vi "Read all flows.vi"(0 "VISA resource name":refnum<visa-resource-name>="COM5") -> (11 "Flow 8":dbl, 13 "Flow 7":dbl, 14 "Flow 1":dbl, 15 "Flow 2":dbl, 16 "Flow 3":dbl, 17 "Flow 4":dbl, 18 "Flow 5":dbl, 19 "Flow 6":dbl)   [LabVIEW 2013]
uses:
  <vilib>/Instr/_visa.llb/VISA Configure Serial Port (Instr).vi
panel:
  out "GCF 8":dbl=1.0
  out "GCF 7":dbl=1.0
  out "GCF 6":dbl=1.0
  out "MFC 8 Size":dbl=1.0
  out "MFC 7 Size":dbl=1.0
  out "MFC 6 Size":dbl=1.0
  out "GCF 5":dbl=0.94
  out "GCF 4":dbl=1.47
  out "GCF 3":dbl=1.22
  out "GCF 2":dbl=0.9
  out "GCF 1":dbl=0.95
  out "MFC 5 Size":dbl=100.0
  out "MFC 4 Size":dbl=50.0
  out "MFC 3 Size":dbl=50.0
  out "MFC 2 Size":dbl=100.0
  out "MFC 1 Size":dbl=50.0
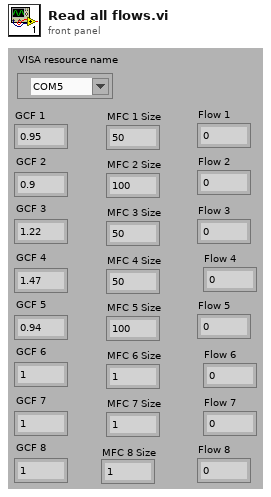
[diagram p1: front panel]
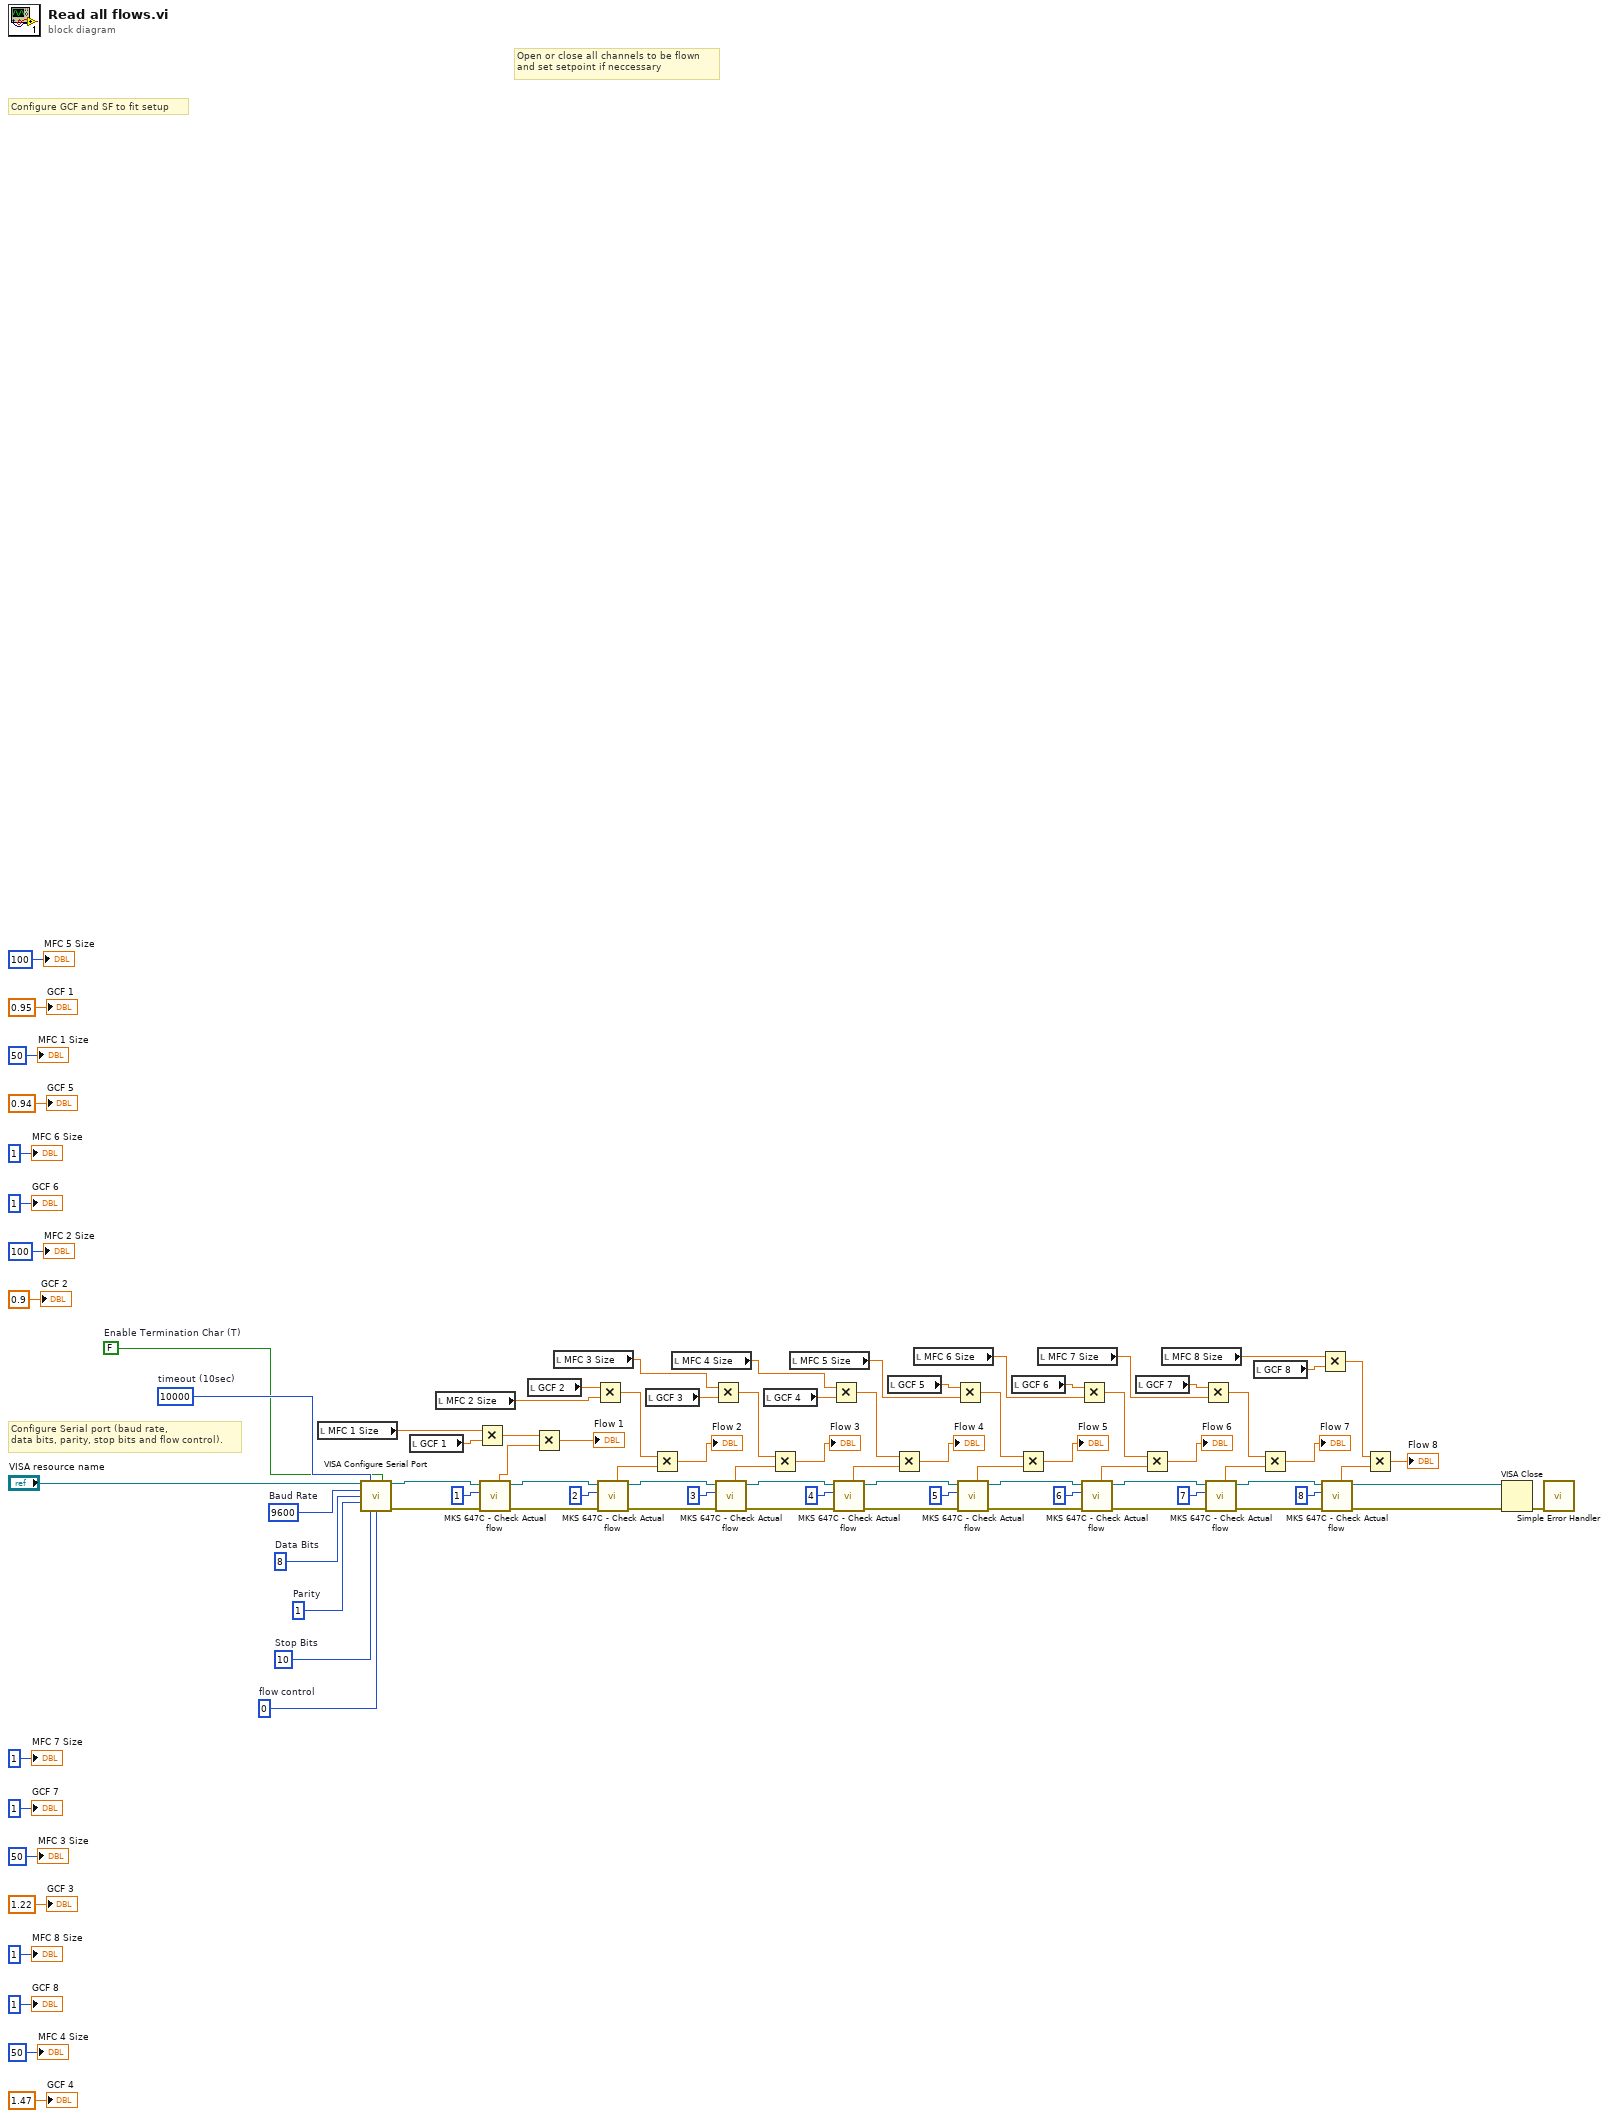
[diagram p0: block diagram]
diagram:
  w84 = 0  # flow control
  w85 = 10  # Stop Bits
  w86 = 1  # Parity
  w87 = 8  # Data Bits
  w88 = 9600  # Baud Rate
  w89 = FALSE  # Enable Termination Char (T)
  w90 = u32 10000  # timeout (10sec)
  # "Open or close all channels to be flown\nand set setpoint if neccessary"
  # "Configure GCF and SF to fit setup"
  # "Configure Serial port (baud rate,\ndata bits, parity, stop bits and flow control)."
  n1 = local read "MFC 1 Size"() -> (w61:dbl)
  n2 = call-poly "VISA Configure Serial Port"("VISA resource name"="VISA resource name", "timeout (10sec)"=w90, "Enable Termination\nChar (T)"=w89, "baud rate (9600)"=w88, "data bits (8)"=w87, "parity (0:none)"=w86, "stop bits (10: 1 bit)"=w85, "flow control (0:none)"=w84) -> ("VISA resource name out"=w66:refnum<visa-resource-name>, "error out"=w64:errorcluster)  [unwired: 6 in]
  n3 = local read "GCF 1"() -> (w60:dbl)
  n4 = local read "MFC 2 Size"() -> (w23:dbl)
  n5 = Multiply(x=w61, y=w60) -> (x*y=w63:dbl)
  n6 = call "MKS 647C - Check Actual flow.vi"("error in (no error)"=w64, "Channel"=1, "VISA resource name (IN)"=w66) -> ("error out"=w36:errorcluster, "VISA resource name (OUT)"=w37:refnum<visa-resource-name>, "Flow value"=w62:dbl)  [unwired: 6 in]
  n7 = local read "GCF 2"() -> (w22:dbl)
  n8 = Multiply(x=w63, y=w62) -> (x*y=→"Flow 1":dbl)
  n9 = local read "MFC 3 Size"() -> (w18:dbl)
  n10 = Multiply(x=w22, y=w23) -> (x*y=w58:dbl)
  n11 = call "MKS 647C - Check Actual flow.vi"("error in (no error)"=w36, "Channel"=2, "VISA resource name (IN)"=w37) -> ("error out"=w35:errorcluster, "VISA resource name (OUT)"=w34:refnum<visa-resource-name>, "Flow value"=w57:dbl)  [unwired: 6 in]
  n12 = local read "GCF 3"() -> (w19:dbl)
  n13 = Multiply(x=w58, y=w57) -> (x*y=→"Flow 2":dbl)
  n14 = local read "MFC 4 Size"() -> (w16:dbl)
  n15 = Multiply(x=w18, y=w19) -> (x*y=w55:dbl)
  n16 = call "MKS 647C - Check Actual flow.vi"("error in (no error)"=w35, "Channel"=3, "VISA resource name (IN)"=w34) -> ("error out"=w32:errorcluster, "VISA resource name (OUT)"=w33:refnum<visa-resource-name>, "Flow value"=w54:dbl)  [unwired: 6 in]
  n17 = local read "GCF 4"() -> (w15:dbl)
  n18 = Multiply(x=w55, y=w54) -> (x*y=→"Flow 3":dbl)
  n19 = local read "MFC 5 Size"() -> (w13:dbl)
  n20 = Multiply(x=w16, y=w15) -> (x*y=w52:dbl)
  n21 = call "MKS 647C - Check Actual flow.vi"("error in (no error)"=w32, "Channel"=4, "VISA resource name (IN)"=w33) -> ("error out"=w24:errorcluster, "VISA resource name (OUT)"=w31:refnum<visa-resource-name>, "Flow value"=w51:dbl)  [unwired: 6 in]
  n22 = local read "GCF 5"() -> (w12:dbl)
  n23 = Multiply(x=w52, y=w51) -> (x*y=→"Flow 4":dbl)
  n24 = local read "MFC 6 Size"() -> (w2:dbl)
  n25 = Multiply(x=w12, y=w13) -> (x*y=w49:dbl)
  n26 = call "MKS 647C - Check Actual flow.vi"("error in (no error)"=w24, "Channel"=5, "VISA resource name (IN)"=w31) -> ("error out"=w30:errorcluster, "VISA resource name (OUT)"=w25:refnum<visa-resource-name>, "Flow value"=w48:dbl)  [unwired: 6 in]
  n27 = local read "GCF 6"() -> (w3:dbl)
  n28 = Multiply(x=w49, y=w48) -> (x*y=→"Flow 5":dbl)
  n29 = local read "MFC 7 Size"() -> (w4:dbl)
  n30 = Multiply(x=w3, y=w2) -> (x*y=w46:dbl)
  n31 = call "MKS 647C - Check Actual flow.vi"("error in (no error)"=w30, "Channel"=6, "VISA resource name (IN)"=w25) -> ("error out"=w29:errorcluster, "VISA resource name (OUT)"=w26:refnum<visa-resource-name>, "Flow value"=w45:dbl)  [unwired: 6 in]
  n32 = local read "GCF 7"() -> (w5:dbl)
  n33 = Multiply(x=w46, y=w45) -> (x*y=→"Flow 6":dbl)
  n34 = local read "MFC 8 Size"() -> (w8:dbl)
  n35 = Multiply(x=w5, y=w4) -> (x*y=w43:dbl)
  n36 = call "MKS 647C - Check Actual flow.vi"("error in (no error)"=w29, "Channel"=7, "VISA resource name (IN)"=w26) -> ("error out"=w28:errorcluster, "VISA resource name (OUT)"=w27:refnum<visa-resource-name>, "Flow value"=w42:dbl)  [unwired: 6 in]
  n37 = local read "GCF 8"() -> (w7:dbl)
  n38 = Multiply(x=w43, y=w42) -> (x*y=→"Flow 7":dbl)
  n39 = Multiply(x=w8, y=w7) -> (x*y=w40:dbl)
  n40 = call "MKS 647C - Check Actual flow.vi"("error in (no error)"=w28, "Channel"=8, "VISA resource name (IN)"=w27) -> ("error out"=w11:errorcluster, "VISA resource name (OUT)"=w10:refnum<visa-resource-name>, "Flow value"=w39:dbl)  [unwired: 6 in]
  n41 = Multiply(x=w40, y=w39) -> (x*y=→"Flow 8":dbl)
  n42 = VISA Close(VISA resource name=w10, error in (no error)=w11) -> (error out=w83:errorcluster)
  n43 = call <vilib>:"Simple Error Handler.vi"("error in (no error)"=w83) -> ()  [unwired: 4 in, 5 out]
  "MFC 1 Size" <- 50
  "GCF 1" <- 0.95
  "MFC 2 Size" <- 100
  "GCF 2" <- 0.9
  "MFC 3 Size" <- 50
  "GCF 3" <- 1.22
  "MFC 4 Size" <- 50
  "GCF 4" <- 1.47
  "MFC 5 Size" <- 100
  "GCF 5" <- 0.94
  "GCF 6" <- 1
  "MFC 6 Size" <- 1
  "MFC 7 Size" <- 1
  "MFC 8 Size" <- 1
  "GCF 7" <- 1
  "GCF 8" <- 1
